vi "Build Robot.vi"(8 "error in":errorcluster, 10 "Robot Elements":T3[](array[typedef])) -> (0 "error out":errorcluster, 1 "Scene Out":refnum<vi>, 2 "Joint Array":T1[](array[typedef]))   [LabVIEW 2017, in "NI_Robotics_3DKinematics.lvlib"]
uses:
  <vilib>/robotics/Kinematics/Plotting/NI_Robotics_3DKinematics.lvlib
  <vilib>/robotics/Kinematics/Plotting/Tree Element.ctl
  <vilib>/robotics/Kinematics/Plotting/Element Type.ctl
  <vilib>/robotics/Kinematics/Plotting/Joint Type.ctl
  <vilib>/robotics/Kinematics/Plotting/Joint Control.ctl
  <vilib>/picture/3D Picture Control/Object/Create Object (name).vi
  <vilib>/picture/3D Picture Control/NI_3D Picture Control.lvlib
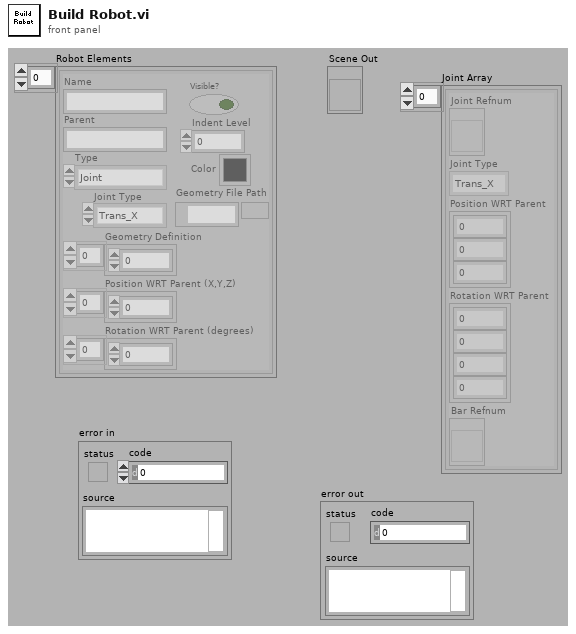
[diagram p1: front panel]
types:
  T1 = typedef "NI_Robotics_3DKinematics.lvlib/Joint Control.ctl" = cluster{"Joint Refnum":refnum<vi>, "Joint Type":T2, "Position WRT Parent":dbl[], "Rotation WRT Parent":dbl[], "Bar Refnum":refnum<vi>}
  T2 = typedef "NI_Robotics_3DKinematics.lvlib/Joint Type.ctl" = enum16{"Trans_X", "Trans_Y", "Trans_Z", "Rot_X", "Rot_Y", "Rot_Z", "None"}
  T3 = typedef "NI_Robotics_3DKinematics.lvlib/Tree Element.ctl" = cluster{"Name":string, "Parent":string, "Type":T4, "Visible?":bool, "Geometry Definition":dbl[], "Position WRT Parent (X,Y,Z)":dbl[], "Rotation WRT Parent (degrees)":dbl[], "Joint Type":T2, "Geometry File Path":path, "Indent Level":i32, "Color":u32}
  T4 = typedef "NI_Robotics_3DKinematics.lvlib/Element Type.ctl" = enum16{"Joint", "Box", "Cylinder", "Cone", "Sphere", "ASE File", "VRML File", "STL File", "Space"}
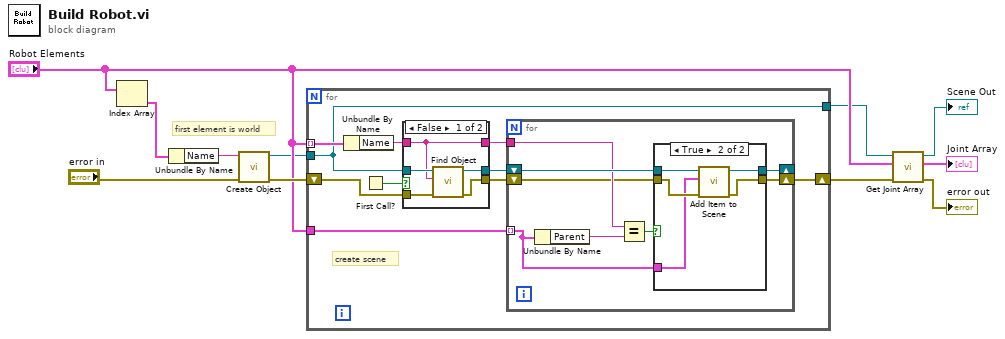
[diagram p0: block diagram]
diagram:
  # "first element is world"
  n1 = Index Array(array="Robot Elements") -> (element=w7:T3)  [unwired: 1 in]
  n2 = Unbundle By Name(w7) -> ("Name"=w3:string)
  n3 = call-poly <vilib>:"Create Object.vi"("error in (no error)"="error in", "Name"=w3) -> ("error out"=w11:errorcluster, "Scene:New Object"=w9:refnum<vi>)  [unwired: 8 in]
  n4 = for {
    tunnel: "Robot Elements" -> [w21]
    tunnel: "Robot Elements" -> [w20] mode=indexing
    shift-right: [w15] -> w5
    shift-left: w11 -> [w14]
    tunnel: [w12] -> w4
    tunnel: w9 -> [w12]
    # "create scene"
    n5 = Unbundle By Name(w20) -> ("Name"=w16:string)
    n6 = First Call?() -> (First Call?: T/F=w19:bool)
    n7 = case shown="False" w19 {
      tunnel: w12 -> [w26 w29]
      tunnel: [w25 w29] -> w18
      tunnel: [w24 w28] -> w17
      tunnel: w16 -> [w24 w28]
      tunnel: w14 -> [w23 w27]
      tunnel: [w22 w27] -> w13
      frame False {
        n8 = call <vilib>:"Find Object.vi"("error in (no error)"=w23, "Object Name"=w24, "Scene Refnum"=w26) -> ("error out"=w22:errorcluster, "Object Refnum"=w25:refnum<vi>)  [unwired: 7 out]
      }
      frame True {
      }
    }
    n9 = for {
      tunnel: w21 -> [w35] mode=indexing
      shift-right: [w30] -> _
      shift-left: w18 -> [w34]
      tunnel: w17 -> [w33]
      shift-right: [w32] -> w15
      shift-left: w13 -> [w31]
      n10 = Unbundle By Name(w35) -> ("Parent"=w37:string)
      n11 = Equal?(x=w33, y=w37) -> (x = y?=w36:bool)
      n12 = case shown="True" w36 {
        tunnel: w34 -> [w39 w44]
        tunnel: w35 -> [_ w40]
        tunnel: [w39 w43] -> w30
        tunnel: [w38 w42] -> w32
        tunnel: w31 -> [w38 w41]
        frame False {
        }
        frame True {
          n13 = call <vilib>:"Add Item to Scene.vi"("error in"=w41, "Tree Element"=w40, "Scene In"=w44) -> ("error out"=w42:errorcluster, "Scene Out"=w43:refnum<vi>)  [unwired: 7 out]
        }
      }
    }
  }
  n14 = call <vilib>:"Get Joint Array.vi"("error in"=w5, "Tree Elements"="Robot Elements", "Scene In"=w4) -> ("error out"=→"error out":errorcluster, "Joint Array"=→"Joint Array":T1[], "Scene Out"=→"Scene Out":refnum<vi>)  [unwired: 6 out]
